vi "LINC Command Global.vi"(0 "item names in":string[](array[string]), 1 "mode":T2, 2 "target name":string, 5 "item formats in":T1[](array[typedef]), 7 "data in":string, 9 "hazardous in":bool, 11 "error in (no error)":errorcluster, 12 "packet name":string, 13 "packet description":string) -> (4 "values out":string[](array[string]), 6 "item formats out":T1[](array[typedef]), 8 "data out":string, 10 "hazardous out":bool[](array[boolean]), 15 "error out":errorcluster)   [LabVIEW 2018, in "STEPkgDriver_LINC.lvlib"]
uses:
  STEPkgDriver_LINC.lvlib
  LINC Format Prototype.ctl
  LINC Global Prototype.ctl
  LINC Global Mode.ctl
  LINC Sim Ops.ctl
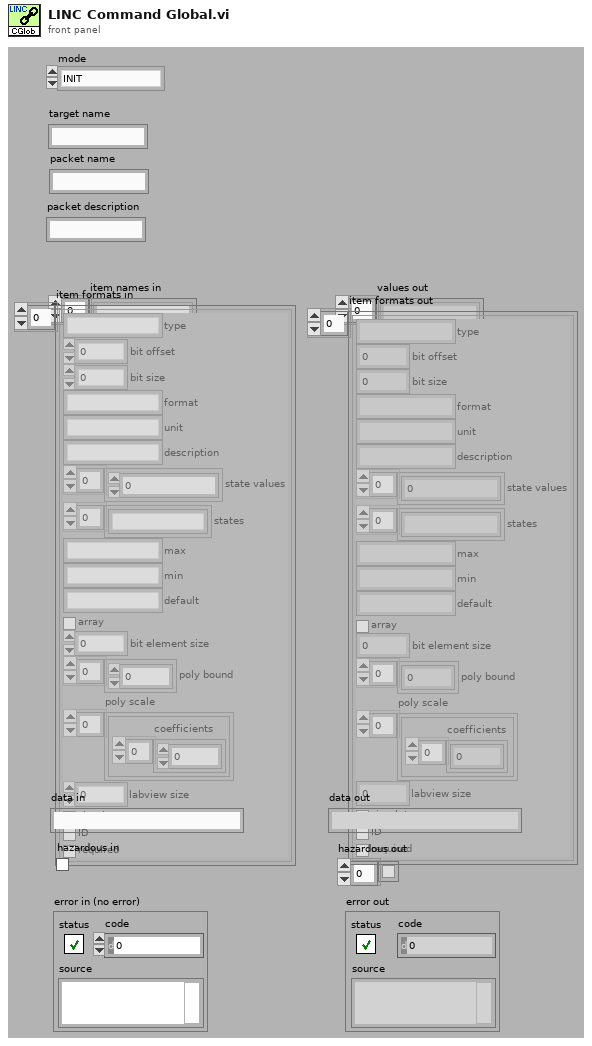
[diagram p1: front panel]
types:
  T1 = typedef "STEPkgDriver_LINC.lvlib/LINC Format Prototype.ctl" = cluster{"type":string, "bit offset":i32, "bit size":i32, "format":string, "unit":string, "description":string, "state values":i64[], "states":string[], "max":string, "min":string, "default":string, "array":bool, "bit element size":i32, "poly bound":dbl[], "poly scale":cluster{"coefficients":dbl[]}[], "labview size":i32, "simulate":bool, "ID":bool, "required":bool}
  T2 = typedef "STEPkgDriver_LINC.lvlib/LINC Global Mode.ctl" = enum16{"INIT", "CLEAR", "ADD_PKT_HDR", "ADD_PKT", "GET_PKT_NAMES", "GET_PKT_DESC", "GET_PKT_HDR", "GET_PKT", "SET_PKT", "SET_DATA", "SIM_EN", "SIM_DS"}
  T3 = typedef "STEPkgDriver_LINC.lvlib/LINC Global Prototype.ctl" = cluster{"packet names":string[], "packet descriptions":string[], "packet hazardous":bool[], "item names":cluster{"names":string[]}[], "item formats":cluster{"formats":T1[], "sim ops":T4[]}[]}
  T4 = typedef "STEPkgDriver_LINC.lvlib/LINC Sim Ops.ctl" = cluster{"byte":i32, "mask":u8}
  T5 = cluster{"item names in":string[], "item formats in":T1[]}
  T6 = cluster{"item formats in":T1[], "sim ops":T4[]}[]
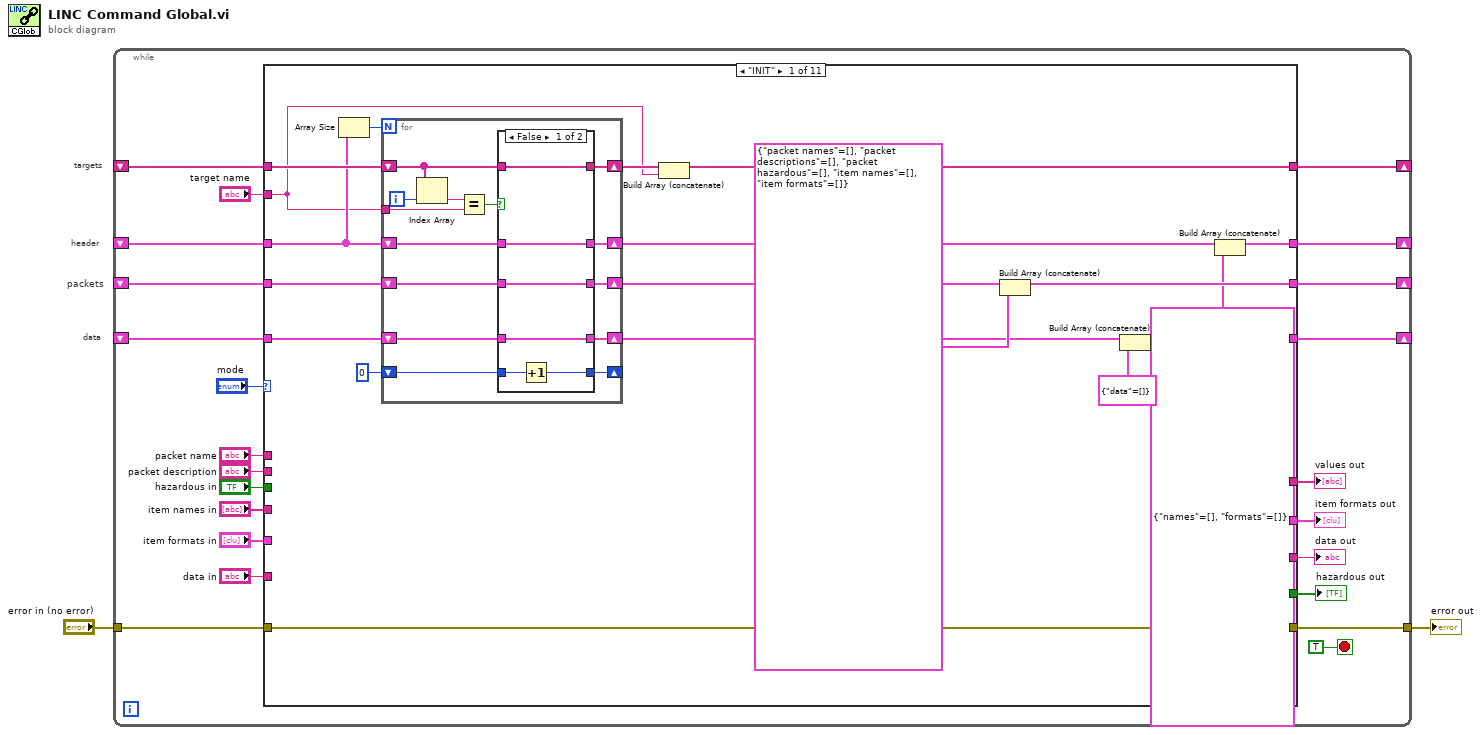
[diagram p0: block diagram]
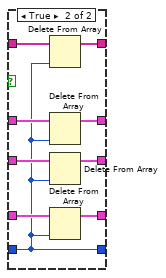
[diagram p2: hidden frame]
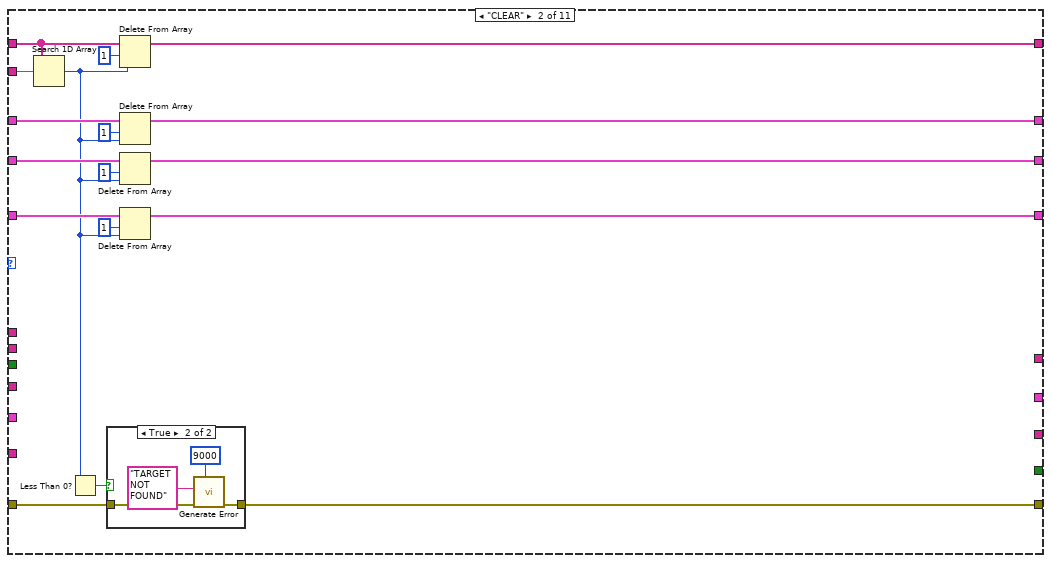
[diagram p3: hidden frame]
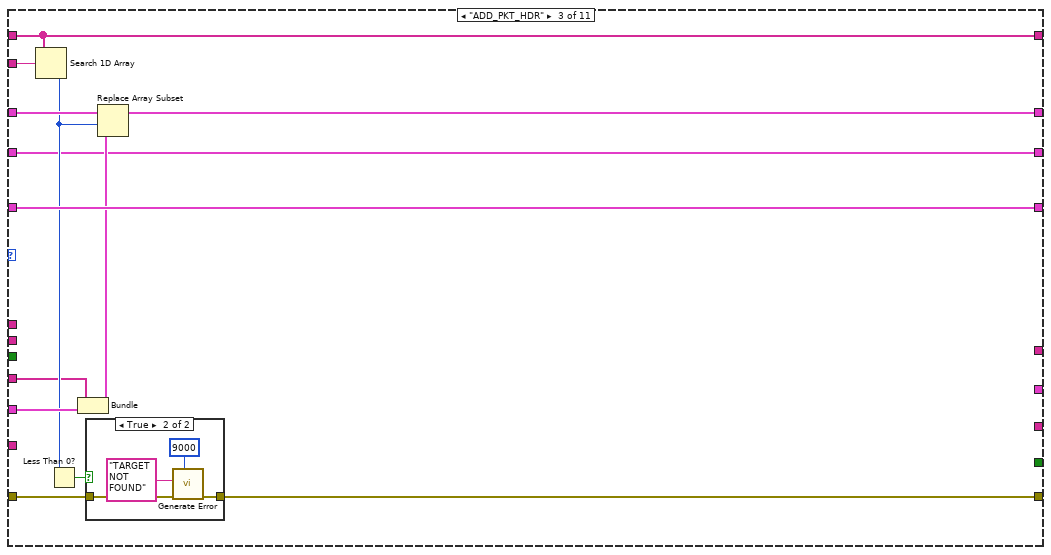
[diagram p5: hidden frame]
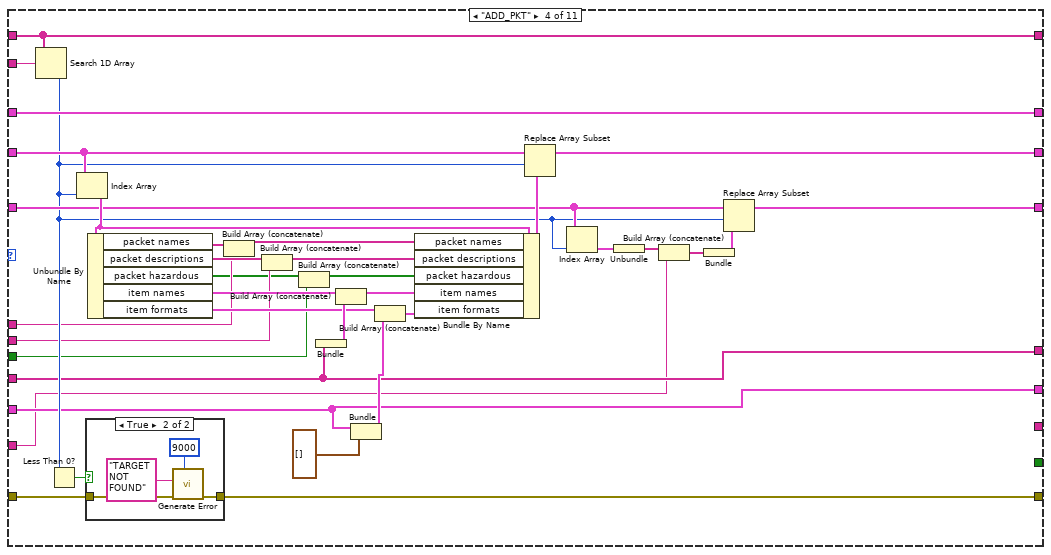
[diagram p7: hidden frame]
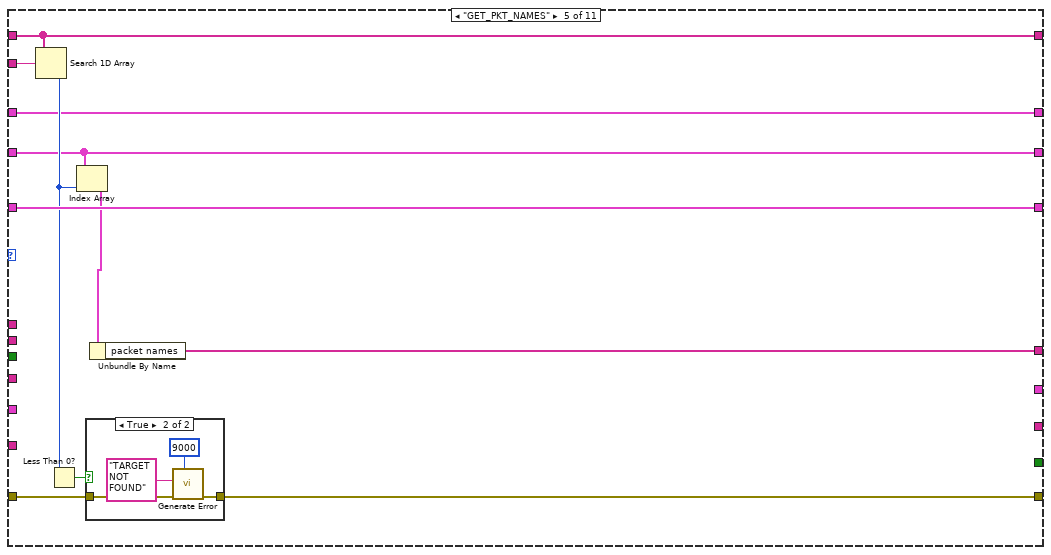
[diagram p9: hidden frame]
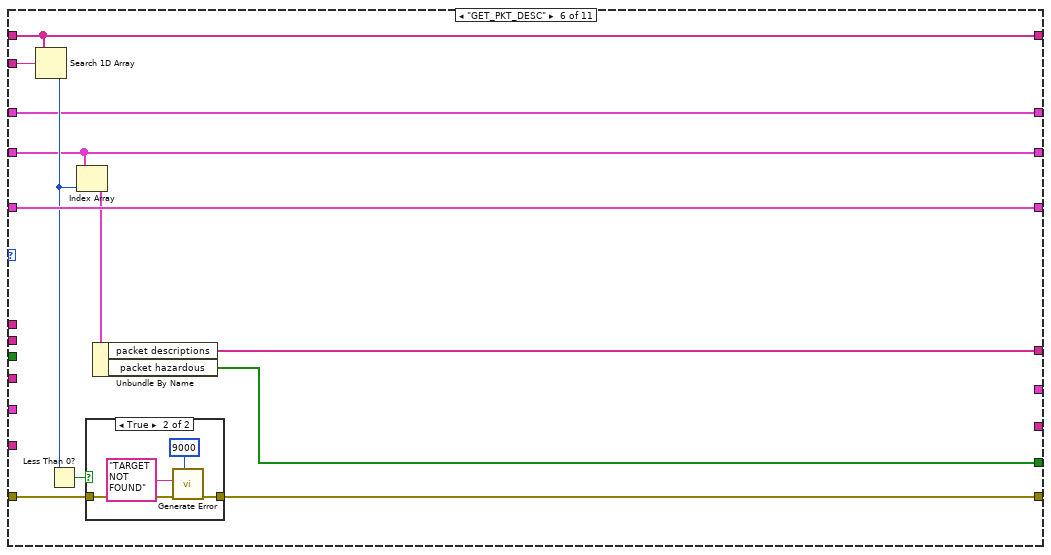
[diagram p11: hidden frame]
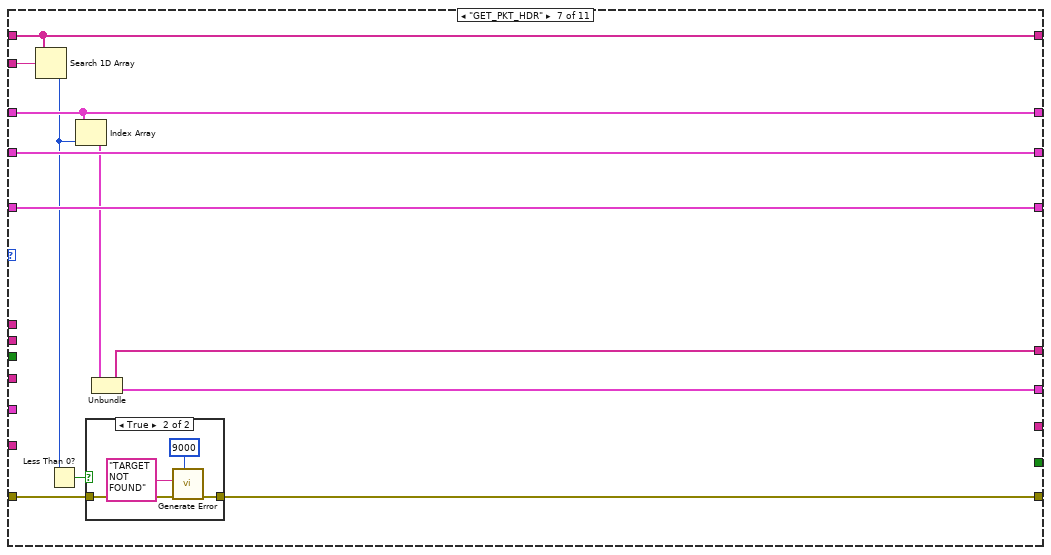
[diagram p13: hidden frame]
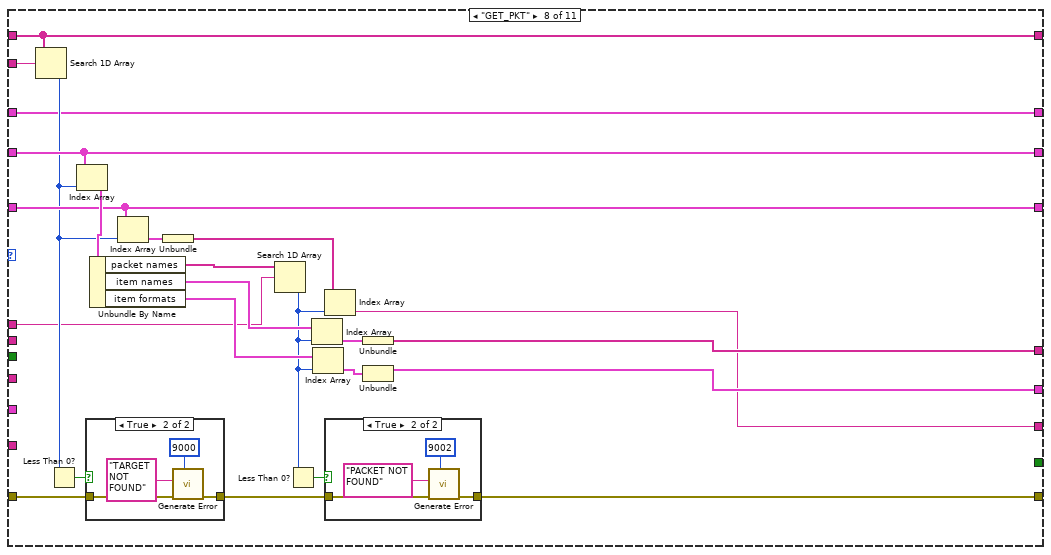
[diagram p15: hidden frame]
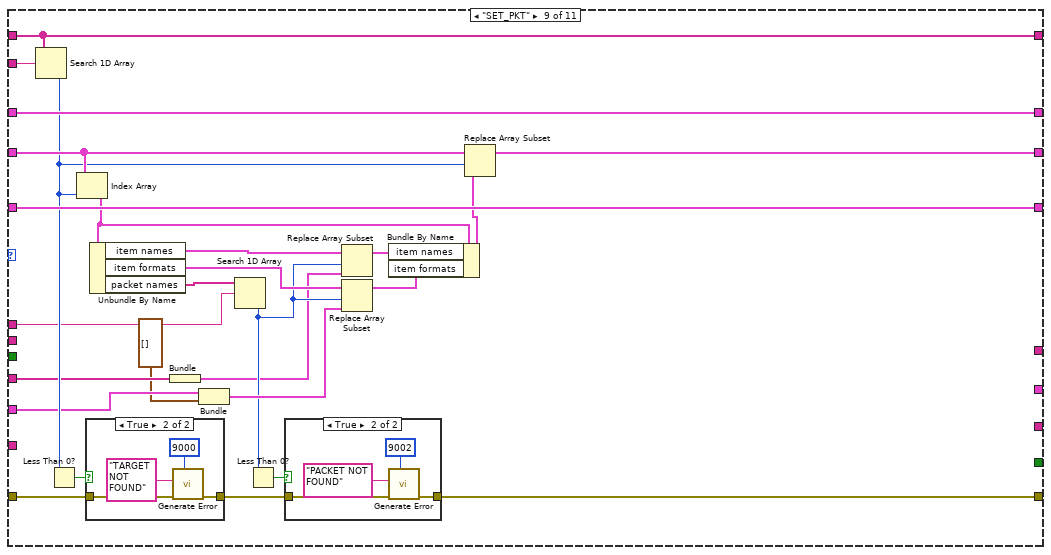
[diagram p18: hidden frame]
diagram:
  # "data"
  # "packets"
  # "header"
  # "targets"
  n1 = while {
    shift-right: [w23] -> _
    shift-left: _ -> [w24]
    shift-right: [w19] -> _
    shift-left: _ -> [w20]
    shift-right: [w17] -> _
    shift-left: _ -> [w18]
    tunnel: "error in (no error)" -> [w10]
    tunnel: [w9] -> w1
    shift-right: [w8] -> _
    shift-left: _ -> [w7]
    stop <- TRUE stop-if-true
    n2 = case shown="\"INIT\"" "mode" {
      selector: "mode" -> [_ _ _ _ _ _ _ _ _ _ w312]
      tunnel: w24 -> [w34 w89 w108 w149 w165 w182 w199 w228 w264 w291 w340]
      tunnel: [w44 w88 w108 w149 w165 w182 w199 w228 w264 w291 w340] -> w23
      tunnel: "target name" -> [w30 w90 w107 w148 w164 w181 w198 w227 w263 w292 w339]
      tunnel: w20 -> [w32 w85 w97 w134 w156 w173 w197 w218 w254 w290 w326]
      tunnel: [w43 w84 w97 w135 w156 w173 w197 w218 w253 w290 w325] -> w19
      tunnel: w18 -> [w29 w82 w102 w129 w163 w180 w194 w212 w256 w288 w316]
      tunnel: [w42 w81 w102 w130 w163 w180 w194 w212 w256 w289 w316] -> w17
      tunnel: "item names in" -> [_ _ w96 w121 _ _ _ _ w245 _ w330]
      tunnel: "item formats in" -> [_ _ w103 w122 _ _ _ _ w247 _ _]
      tunnel: [_ _ _ w121 w157 w174 w188 w220 _ _ w318] -> w14
      tunnel: [_ _ _ w122 _ _ w189 w219 _ _ w319] -> w13
      tunnel: [_ _ _ _ _ _ _ w208 _ _ w313] -> w12
      tunnel: "data in" -> [_ _ _ w120 _ _ _ _ _ w284 _]
      tunnel: w10 -> [w39 w79 w105 w132 w160 w177 w195 w216 w260 w280 w333]
      tunnel: [w39 w78 w104 w125 w158 w175 w190 w213 w257 w279 w321] -> w9
      tunnel: w7 -> [w31 w76 w101 w124 w155 w172 w193 w207 w255 w276 w309]
      tunnel: [w38 w74 w100 w124 w155 w172 w193 w207 w255 w276 w309] -> w8
      tunnel: "packet name" -> [_ _ _ w119 _ _ _ w206 w240 w275 w307]
      tunnel: "packet description" -> [_ _ _ w118 _ _ _ _ _ _ _]
      tunnel: "hazardous in" -> [_ _ _ w115 _ _ _ _ _ _ _]
      tunnel: [_ _ _ _ _ w171 _ _ _ _ _] -> w3
      frame "INIT" {
        n3 = Array Size(array=w31) -> (size(s)=w36:i32)
        n4 = for {
          N: w36 -> [_]
          shift-right: [w51] -> w33
          shift-left: w34 -> [w57]
          shift-right: [w50] -> w28
          shift-left: w31 -> [w56]
          shift-right: [w49] -> w27
          shift-left: w32 -> [w55]
          tunnel: w30 -> [w53]
          shift-right: [w47] -> _
          shift-left: 0 -> [w48]
          shift-right: [w45] -> w26
          shift-left: w29 -> [w46]
          i -> [w58]
          n5 = Index Array(array=w57, index=w58) -> (element=w54:string)
          n6 = Equal?(x=w54, y=w53) -> (x = y?=w52:bool)
          n7 = case shown="False" w52 {
            tunnel: w57 -> [w64 w73]
            tunnel: w56 -> [w63 w71]
            tunnel: w55 -> [w62 w70]
            tunnel: [w64 w72] -> w51
            tunnel: [w63 w69] -> w50
            tunnel: [w62 w68] -> w49
            tunnel: w48 -> [w61 w66]
            tunnel: [w60 w66] -> w47
            tunnel: w46 -> [w59 w67]
            tunnel: [w59 w65] -> w45
            frame False {
              n8 = Increment(x=w61) -> (x+1=w60:i32)
            }
            frame True {
              n9 = Delete From Array(array=w73, index=w66) -> (array with subset deleted=w72:string[])  [unwired: 1 in, 1 out]
              n10 = Delete From Array(array=w71, index=w66) -> (array with subset deleted=w69:cluster{"names":string[], "formats":T1[]}[])  [unwired: 1 in, 1 out]
              n11 = Delete From Array(array=w70, index=w66) -> (array with subset deleted=w68:T3[])  [unwired: 1 in, 1 out]
              n12 = Delete From Array(array=w67, index=w66) -> (array with subset deleted=w65:cluster{"data":string[]}[])  [unwired: 1 in, 1 out]
            }
          }
        }
        n13 = Build Array (concatenate)(w33, w30) -> (w44:string[])
        n14 = Build Array (concatenate)(w27, T3 {"packet names"=[], "packet descriptions"=[], "packet hazardous"=[], "item names"=[], "item formats"=[]} ("housekeeping")) -> (w43:T3[])
        n15 = Build Array (concatenate)(w26, cluster{"data":string[]} {"data"=[]} ("data")) -> (w42:cluster{"data":string[]}[])
        n16 = Build Array (concatenate)(w28, cluster{"names":string[], "formats":T1[]} {"names"=[], "formats"=[]}) -> (w38:cluster{"names":string[], "formats":T1[]}[])
      }
      frame "CLEAR" {
        n17 = Search 1D Array(1D array=w89, element=w90) -> (index of element=w75:i32)  [unwired: 1 in]
        n18 = Less Than 0?(x=w75) -> (x < 0?=w80:bool)
        n19 = case shown="True" w80 {
          tunnel: w79 -> [w91 w95]
          tunnel: [w91 w94] -> w78
          frame False {
          }
          frame True {
            n20 = call "Generate Error.vi"("error code (-1301)"=9000, "error in"=w95, "description"="TARGET NOT FOUND") -> ("error out"=w94:errorcluster)  [unwired: 8 in]
          }
        }
        n21 = Delete From Array(array=w89, length=1, index=w75) -> (array with subset deleted=w88:string[])  [unwired: 1 out]
        n22 = Delete From Array(array=w76, length=1, index=w75) -> (array with subset deleted=w74:cluster{"names":string[], "formats":T1[]}[])  [unwired: 1 out]
        n23 = Delete From Array(array=w85, length=1, index=w75) -> (array with subset deleted=w84:T3[])  [unwired: 1 out]
        n24 = Delete From Array(array=w82, length=1, index=w75) -> (array with subset deleted=w81:cluster{"data":string[]}[])  [unwired: 1 out]
      }
      frame "ADD_PKT_HDR" {
        n25 = Search 1D Array(1D array=w108, element=w107) -> (index of element=w99:i32)  [unwired: 1 in]
        n26 = Less Than 0?(x=w99) -> (x < 0?=w106:bool)
        n27 = Bundle("item names in"=w96, "item formats in"=w103) -> (w98:T5)  [unwired: 1 in]
        n28 = case shown="True" w106 {
          tunnel: w105 -> [w109 w113]
          tunnel: [w109 w112] -> w104
          frame False {
          }
          frame True {
            n29 = call "Generate Error.vi"("error code (-1301)"=9000, "error in"=w113, "description"="TARGET NOT FOUND") -> ("error out"=w112:errorcluster)  [unwired: 8 in]
          }
        }
        n30 = Replace Array Subset(array=w101, new element=w98, index=w99) -> (w100:cluster{"names":string[], "formats":T1[]}[])
      }
      frame "ADD_PKT" {
        n31 = Search 1D Array(1D array=w149, element=w148) -> (index of element=w123:i32)  [unwired: 1 in]
        n32 = Less Than 0?(x=w123) -> (x < 0?=w133:bool)
        n33 = Index Array(array=w134, index=w123) -> (element=w141:T3)
        n34 = case shown="True" w133 {
          tunnel: w132 -> [w150 w154]
          tunnel: [w150 w153] -> w125
          frame False {
          }
          frame True {
            n35 = call "Generate Error.vi"("error code (-1301)"=9000, "error in"=w154, "description"="TARGET NOT FOUND") -> ("error out"=w153:errorcluster)  [unwired: 8 in]
          }
        }
        n36 = Unbundle By Name(w141) -> ("packet names"=w147:string[], "packet descriptions"=w146:string[], "packet hazardous"=w117:bool[], "item names"=w145:cluster{"names":string[]}[], "item formats"=w143:cluster{"formats":T1[], "sim ops":T4[]}[])
        n37 = Build Array (concatenate)(w147, w119) -> (w140:string[])
        n38 = Build Array (concatenate)(w146, w118) -> (w139:string[])
        n39 = Build Array (concatenate)(w117, w115) -> (w116:bool[])
        n40 = Bundle("item names in"=w121) -> (w144:cluster{"item names in":string[]})  [unwired: 1 in]
        n41 = Build Array (concatenate)(w145, w144) -> (w138:cluster{"item names in":string[]}[])
        n42 = Bundle("item formats in"=w122, "sim ops"=T4[] []) -> (w142:cluster{"item formats in":T1[], "sim ops":T4[]})  [unwired: 1 in]
        n43 = Build Array (concatenate)(w143, w142) -> (w137:T6)
        n44 = Bundle By Name(cluster=w141, "packet names"=w140, "packet descriptions"=w139, "packet hazardous"=w116, "item names"=w138, "item formats"=w137) -> (w136:T3)
        n45 = Replace Array Subset(array=w134, new element=w136, index=w123) -> (w135:T3[])
        n46 = Index Array(array=w129, index=w123) -> (element=w128:cluster{"data":string[]})
        n47 = Unbundle(w128) -> ("data"=w127:string[])
        n48 = Build Array (concatenate)(w127, w120) -> (w126:string[])
        n49 = Bundle(w126) -> (w131:cluster{string[]})  [unwired: 1 in]
        n50 = Replace Array Subset(array=w129, new element=w131, index=w123) -> (w130:cluster{"data":string[]}[])
      }
      frame "GET_PKT_NAMES" {
        n51 = Search 1D Array(1D array=w165, element=w164) -> (index of element=w159:i32)  [unwired: 1 in]
        n52 = Less Than 0?(x=w159) -> (x < 0?=w161:bool)
        n53 = Index Array(array=w156, index=w159) -> (element=w162:T3)
        n54 = case shown="True" w161 {
          tunnel: w160 -> [w166 w170]
          tunnel: [w166 w169] -> w158
          frame False {
          }
          frame True {
            n55 = call "Generate Error.vi"("error code (-1301)"=9000, "error in"=w170, "description"="TARGET NOT FOUND") -> ("error out"=w169:errorcluster)  [unwired: 8 in]
          }
        }
        n56 = Unbundle By Name(w162) -> ("packet names"=w157:string[])
      }
      frame "GET_PKT_DESC" {
        n57 = Search 1D Array(1D array=w182, element=w181) -> (index of element=w176:i32)  [unwired: 1 in]
        n58 = Less Than 0?(x=w176) -> (x < 0?=w178:bool)
        n59 = Index Array(array=w173, index=w176) -> (element=w179:T3)
        n60 = case shown="True" w178 {
          tunnel: w177 -> [w183 w187]
          tunnel: [w183 w186] -> w175
          frame False {
          }
          frame True {
            n61 = call "Generate Error.vi"("error code (-1301)"=9000, "error in"=w187, "description"="TARGET NOT FOUND") -> ("error out"=w186:errorcluster)  [unwired: 8 in]
          }
        }
        n62 = Unbundle By Name(w179) -> ("packet descriptions"=w174:string[], "packet hazardous"=w171:bool[])
      }
      frame "GET_PKT_HDR" {
        n63 = Search 1D Array(1D array=w199, element=w198) -> (index of element=w192:i32)  [unwired: 1 in]
        n64 = Less Than 0?(x=w192) -> (x < 0?=w196:bool)
        n65 = Index Array(array=w193, index=w192) -> (element=w191:cluster{"names":string[], "formats":T1[]})
        n66 = case shown="True" w196 {
          tunnel: w195 -> [w200 w204]
          tunnel: [w200 w203] -> w190
          frame False {
          }
          frame True {
            n67 = call "Generate Error.vi"("error code (-1301)"=9000, "error in"=w204, "description"="TARGET NOT FOUND") -> ("error out"=w203:errorcluster)  [unwired: 8 in]
          }
        }
        n68 = Unbundle(w191) -> ("names"=w188:string[], "formats"=w189:T1[])
      }
      frame "GET_PKT" {
        n69 = Search 1D Array(1D array=w228, element=w227) -> (index of element=w211:i32)  [unwired: 1 in]
        n70 = Less Than 0?(x=w211) -> (x < 0?=w217:bool)
        n71 = Index Array(array=w218, index=w211) -> (element=w226:T3)
        n72 = case shown="True" w217 {
          tunnel: w216 -> [w234 w238]
          tunnel: [w234 w237] -> w214
          frame False {
          }
          frame True {
            n73 = call "Generate Error.vi"("error code (-1301)"=9000, "error in"=w238, "description"="TARGET NOT FOUND") -> ("error out"=w237:errorcluster)  [unwired: 8 in]
          }
        }
        n74 = Unbundle By Name(w226) -> ("packet names"=w225:string[], "item names"=w224:cluster{"names":string[]}[], "item formats"=w223:cluster{"formats":T1[], "sim ops":T4[]}[])
        n75 = Index Array(array=w212, index=w211) -> (element=w210:cluster{"data":string[]})
        n76 = Unbundle(w210) -> ("data"=w209:string[])
        n77 = Search 1D Array(1D array=w225, element=w206) -> (index of element=w205:i32)  [unwired: 1 in]
        n78 = Less Than 0?(x=w205) -> (x < 0?=w215:bool)
        n79 = Index Array(array=w224, index=w205) -> (element=w222:cluster{"names":string[]})
        n80 = Index Array(array=w223, index=w205) -> (element=w221:cluster{"formats":T1[], "sim ops":T4[]})
        n81 = Index Array(array=w209, index=w205) -> (element=w208:string)
        n82 = case shown="True" w215 {
          tunnel: w214 -> [w229 w233]
          tunnel: [w229 w232] -> w213
          frame False {
          }
          frame True {
            n83 = call "Generate Error.vi"("error code (-1301)"=9002, "error in"=w233, "description"="PACKET NOT FOUND") -> ("error out"=w232:errorcluster)  [unwired: 8 in]
          }
        }
        n84 = Unbundle(w222) -> ("names"=w220:string[])
        n85 = Unbundle(w221) -> ("formats"=w219:T1[])  [unwired: 1 out]
      }
      frame "SET_PKT" {
        n86 = Search 1D Array(1D array=w264, element=w263) -> (index of element=w252:i32)  [unwired: 1 in]
        n87 = Less Than 0?(x=w252) -> (x < 0?=w261:bool)
        n88 = Index Array(array=w254, index=w252) -> (element=w250:T3)
        n89 = case shown="True" w261 {
          tunnel: w260 -> [w270 w274]
          tunnel: [w270 w273] -> w258
          frame False {
          }
          frame True {
            n90 = call "Generate Error.vi"("error code (-1301)"=9000, "error in"=w274, "description"="TARGET NOT FOUND") -> ("error out"=w273:errorcluster)  [unwired: 8 in]
          }
        }
        n91 = Unbundle By Name(w250) -> ("item names"=w244:cluster{"names":string[]}[], "item formats"=w251:cluster{"formats":T1[], "sim ops":T4[]}[], "packet names"=w262:string[])
        n92 = Bundle("item names in"=w245) -> (w241:cluster{"item names in":string[]})  [unwired: 1 in]
        n93 = Bundle("item formats in"=w247, "sim ops"=T4[] []) -> (w246:cluster{"item formats in":T1[], "sim ops":T4[]})  [unwired: 1 in]
        n94 = Search 1D Array(1D array=w262, element=w240) -> (index of element=w242:i32)  [unwired: 1 in]
        n95 = Less Than 0?(x=w242) -> (x < 0?=w259:bool)
        n96 = case shown="True" w259 {
          tunnel: w258 -> [w265 w269]
          tunnel: [w265 w268] -> w257
          frame False {
          }
          frame True {
            n97 = call "Generate Error.vi"("error code (-1301)"=9002, "error in"=w269, "description"="PACKET NOT FOUND") -> ("error out"=w268:errorcluster)  [unwired: 8 in]
          }
        }
        n98 = Replace Array Subset(array=w244, new element=w241, index=w242) -> (w243:cluster{"names":string[]}[])
        n99 = Replace Array Subset(array=w251, new element=w246, index=w242) -> (w249:cluster{"formats":T1[], "sim ops":T4[]}[])
        n100 = Bundle By Name(cluster=w250, "item names"=w243, "item formats"=w249) -> (w248:T3)
        n101 = Replace Array Subset(array=w254, new element=w248, index=w252) -> (w253:T3[])
      }
      frame "SET_DATA" {
        n102 = Search 1D Array(1D array=w291, element=w292) -> (index of element=w278:i32)  [unwired: 1 in]
        n103 = Less Than 0?(x=w278) -> (x < 0?=w283:bool)
        n104 = Index Array(array=w290, index=w278) -> (element=w295:T3)
        n105 = case shown="True" w283 {
          tunnel: w280 -> [w301 w305]
          tunnel: [w301 w304] -> w281
          frame False {
          }
          frame True {
            n106 = call "Generate Error.vi"("error code (-1301)"=9000, "error in"=w305, "description"="TARGET NOT FOUND") -> ("error out"=w304:errorcluster)  [unwired: 8 in]
          }
        }
        n107 = Unbundle By Name(w295) -> ("packet names"=w294:string[])
        n108 = Index Array(array=w288, index=w278) -> (element=w293:cluster{"data":string[]})
        n109 = Unbundle(w293) -> ("data"=w287:string[])
        n110 = Search 1D Array(1D array=w294, element=w275) -> (index of element=w277:i32)  [unwired: 1 in]
        n111 = Less Than 0?(x=w277) -> (x < 0?=w282:bool)
        n112 = Replace Array Subset(array=w287, new element=w284, index=w277) -> (w286:string[])
        n113 = case shown="True" w282 {
          tunnel: w281 -> [w296 w300]
          tunnel: [w296 w299] -> w279
          frame False {
          }
          frame True {
            n114 = call "Generate Error.vi"("error code (-1301)"=9002, "error in"=w300, "description"="PACKET NOT FOUND") -> ("error out"=w299:errorcluster)  [unwired: 8 in]
          }
        }
        n115 = Bundle("data"=w286) -> (w285:cluster{"data":string[]})  [unwired: 1 in]
        n116 = Replace Array Subset(array=w288, new element=w285, index=w278) -> (w289:cluster{"data":string[]}[])
      }
      frame "SIM_EN", "SIM_DS" {
        n117 = Equal?(x=w312, y=LINC_Global_Mode."SIM_EN" ("mode")) -> (x = y?=w311:bool)
        n118 = Search 1D Array(1D array=w340, element=w339) -> (index of element=w315:i32)  [unwired: 1 in]
        n119 = Less Than 0?(x=w315) -> (x < 0?=w334:bool)
        n120 = Index Array(array=w326, index=w315) -> (element=w324:T3)
        n121 = case shown="True" w334 {
          tunnel: w333 -> [w362 w366]
          tunnel: [w362 w365] -> w331
          frame False {
          }
          frame True {
            n122 = call "Generate Error.vi"("error code (-1301)"=9000, "error in"=w366, "description"="TARGET NOT FOUND") -> ("error out"=w365:errorcluster)  [unwired: 8 in]
          }
        }
        n123 = Unbundle By Name(w324) -> ("packet names"=w338:string[], "item names"=w337:cluster{"names":string[]}[], "item formats"=w327:cluster{"formats":T1[], "sim ops":T4[]}[])
        n124 = Index Array(array=w316, index=w315) -> (element=w317:cluster{"data":string[]})
        n125 = Unbundle(w317) -> ("data"=w314:string[])
        n126 = Search 1D Array(1D array=w338, element=w307) -> (index of element=w310:i32)  [unwired: 1 in]
        n127 = Less Than 0?(x=w310) -> (x < 0?=w332:bool)
        n128 = Index Array(array=w314, index=w310) -> (element=w313:string)
        n129 = Index Array(array=w337, index=w310) -> (element=w336:cluster{"names":string[]})
        n130 = Index Array(array=w327, index=w310) -> (element=w335:cluster{"formats":T1[], "sim ops":T4[]})
        n131 = case shown="True" w332 {
          tunnel: w331 -> [w357 w361]
          tunnel: [w357 w360] -> w322
          frame False {
          }
          frame True {
            n132 = call "Generate Error.vi"("error code (-1301)"=9002, "error in"=w361, "description"="PACKET NOT FOUND") -> ("error out"=w360:errorcluster)  [unwired: 8 in]
          }
        }
        n133 = Unbundle(w336) -> ("names"=w318:string[])
        n134 = Unbundle(w335) -> ("formats"=w329:T1[])  [unwired: 1 out]
        n135 = for {
          tunnel: w318 -> [w351]
          tunnel: w330 -> [w350] mode=indexing
          shift-right: [w347] -> w319
          shift-left: w329 -> [w348]
          shift-right: [w345] -> w321
          shift-left: w322 -> [w344]
          tunnel: w311 -> [w341]
          n136 = Search 1D Array(1D array=w351, element=w350) -> (index of element=w343:i32)  [unwired: 1 in]
          n137 = Less Than 0?(x=w343) -> (x < 0?=w342:bool)
          n138 = Index Array(array=w348, index=w343) -> (element=w349:T1)
          n139 = Bundle By Name(cluster=w349, "simulate"=w341) -> (w346:T1)
          n140 = Replace Array Subset(array=w348, new element=w346, index=w343) -> (w347:T1[])
          n141 = case shown="True" w342 {
            tunnel: w344 -> [w352 w356]
            tunnel: [w352 w355] -> w345
            frame False {
            }
            frame True {
              n142 = call "Generate Error.vi"("error code (-1301)"=9003, "error in"=w356, "description"="ITEM NOT FOUND") -> ("error out"=w355:errorcluster)  [unwired: 8 in]
            }
          }
        }
        n143 = Bundle("formats"=w319, "sim ops"=T4[] []) -> (w328:cluster{"formats":T1[], "sim ops":T4[]})  [unwired: 1 in]
        n144 = Replace Array Subset(array=w327, new element=w328, index=w310) -> (w320:cluster{"formats":T1[], "sim ops":T4[]}[])
        n145 = Bundle By Name(cluster=w324, "item formats"=w320) -> (w323:T3)
        n146 = Replace Array Subset(array=w326, new element=w323, index=w315) -> (w325:T3[])
      }
    }
    "values out" <- w14
    "item formats out" <- w13
    "data out" <- w12
    "hazardous out" <- w3
  }
  "error out" <- w1
